vi "Callback - Set Value.vi"(10 "Value":dbl, 11 "Number Widget in":refnum<class "LQObject.lvclass">) -> ()   [LabVIEW 2014, in "6. Reusing Components Dynamically.lvlib" / "Number Widget.lvclass"]
doc: "A callback VI, designed to set the value of a Number Widget when a numeric signal is emitted.\n\n\nCopyright (c) 2019 Sze Howe Koh.\nThis code is licensed under the MIT license."
uses:
  Number Widget.lvclass
  <vilib>/addons/LQ/LQ Core/LQObject/LQObject.lvclass
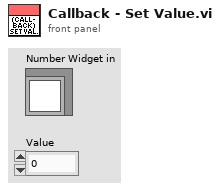
[diagram p1: front panel]
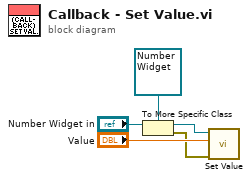
[diagram p0: block diagram]
diagram:
  n1 = To More Specific Class(target class=refnum<class "Number Widget.lvclass"> refnum ("Number Widget"), reference="Number Widget in") -> (specific class reference=w3:refnum<class "Number Widget.lvclass">, error out=w1:errorcluster)  [unwired: 1 in]
  n2 = call "Set Value.vi"("Error In"=w1, "Value"="Value", "Number Widget In"=w3) -> ()  [unwired: 7 in, 2 out]
